vi "svl_Exp Avg Level with IC (final value)_octave.vi"(0 "scaled signal [EU]":dbl[](array[numeric]) format="%.2f", 1 "time constant [ms]":dbl=125.0 min=0.0 format="%.2f", 2 "sampling frequency [Hz]":dbl=10000.0 format="%.2f", 3 "exponential mode":enum16{"Slow", "Fast", "Impulse", "Custom"}(ring)=enum."Fast", 4 "init/cont (init:F)":bool, 5 "initial filter state":T1 {"peak detector" format="%.2f"; "exponential averaging" format="%.2f"}) -> (6 "exp avg [EU^2 rms] (final value)":dbl format="%.2f", 7 "actual time constant [ms]":dbl=125.0 format="%.2f", 8 "final filter state":T1 {"peak detector" format="%.2f"; "exponential averaging" format="%.2f"})   [LabVIEW 2017]
doc: "Computes the exponential averaged level of the input signal X based on the selected exponential averaging mode and returns only the last value of this level.\nThe initial filter state and the final filter state parameters keep track of the internal state of the filter to ensure continuous operation of the filter if continuous mode is used."
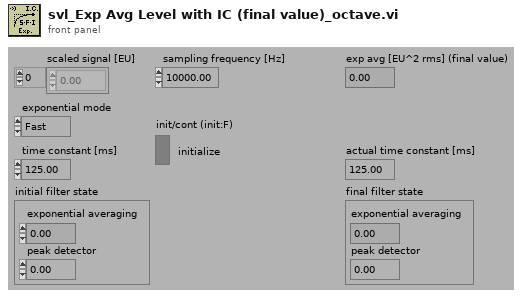
[diagram p1: front panel]
types:
  T1 = cluster{"exponential averaging":dbl, "peak detector":dbl}
  T2 = cluster{"Reverse Coefficients":dbl[], "Forward Coefficients":dbl[]}
  T3 = cluster{"final filter state":dbl, "final filter state":dbl}
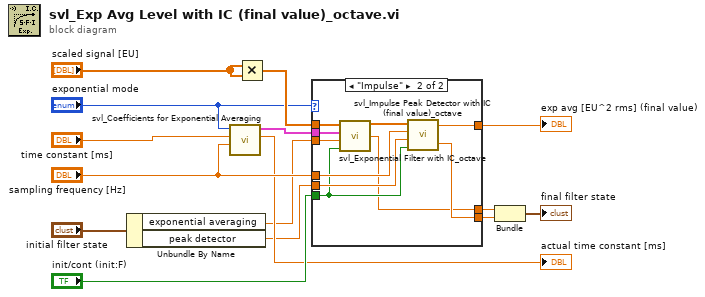
[diagram p0: block diagram]
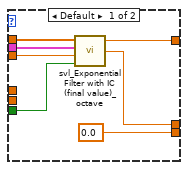
[diagram p2: hidden frame]
diagram:
  n1 = Unbundle By Name("initial filter state") -> ("exponential averaging"=w6:dbl, "peak detector"=w5:dbl)
  n2 = call <vilib>:"svl_Coefficients for Exponential Averaging.vi"("sampling frequency [Hz]"="sampling frequency [Hz]", "time constant [ms]"="time constant [ms]", "exponential mode"="exponential mode") -> ("actual time constant [ms]"=→"actual time constant [ms]":dbl, "filter coefficients"=w14:T2)  [unwired: 3 in]
  n3 = Multiply(x="scaled signal [EU]", y="scaled signal [EU]") -> (x*y=w12:dbl[])
  n4 = case shown="\"Impulse\"" "exponential mode" {
    tunnel: w14 -> [w20 w26]
    tunnel: "init/cont (init:F)" -> [w18 w24]
    tunnel: w6 -> [w19 w25]
    tunnel: w12 -> [w21 w27]
    tunnel: "sampling frequency [Hz]" -> [_ w32]
    tunnel: w5 -> [_ w31]
    tunnel: [w17 w23] -> w4
    tunnel: [0.0 ("Final condition") w30] -> w3
    tunnel: [w16 w29] -> w1
    frame Default {
      n5 = call <vilib>:"svl_Exponential Filter with IC (final value)_octave.vi"("init/cont (init:F)"=w18, "initial filter state"=w19, "filter coefficients"=w20, "X"=w21) -> ("final filter state"=w17:dbl, "filtered X (final value)"=w16:dbl)  [unwired: 1 out]
    }
    frame "Impulse" {
      n6 = call <vilib>:"svl_Exponential Filter with IC_octave.vi"("init/cont (init:F)"=w24, "initial filter state"=w25, "filter coefficients"=w26, "X"=w27) -> ("final filter state"=w23:dbl, "filtered X"=w28:dbl[])  [unwired: 1 out]
      n7 = call <vilib>:"svl_Impulse Peak Detector with IC (final value)_octave.vi"("init/cont (init:F)"=w24, "initial filter state"=w31, "sampling frequency [Hz]"=w32, "X"=w28) -> ("final filter state"=w30:dbl, "filtered X (final value)"=w29:dbl)
    }
  }
  "exp avg [EU^2 rms] (final value)" <- w1
  n8 = Bundle("final filter state"=w4, "final filter state"=w3) -> (→"final filter state":T3)  [unwired: 1 in]
